vi "GDSAPI_CreateInterface.vi"(7 "KeepLvClassRefOpen(False)":bool, 8 "error in (no error)":errorcluster, 9 "ClassIcon(Random colors are used if not wired)":T1, 10 "CreateInterfaceType":T3, 11 "ProjectItemToCreateClassUnder":refnum<vi>) -> (0 "error out":errorcluster, 2 "LVClassLibraryRefnum":refnum<vi>, 3 "LvClassFileOut":path)   [LabVIEW 2020]
doc: "NOT Yet implemented"
uses:
  ClassProviders/Provider_LvNativeClass/ClassWriterNative_class/ClassWriterNative.lvclass
  ClassProviders/Common/LvIcon_class/GDSLvIcon_ClassColorTypes.ctl
  ClassProviders/Common/CommonVIs/CommonVIs_AttributeDataType.ctl
  ClassProviders/Common/String/GDSString_AccessScopeModifierType.ctl
  ClassProviders/Common/CommonVIs/CommonVIs_AttributeType.ctl
  ClassProviders/Provider_BaseClassInterface/ClassWriter_class/InterfaceMethodsToCreate.ctl
  ClassProviders/Provider_BaseClassInterface/ClassWriter_class/ClassWriter.lvclass
  ClassProviders/Provider_BaseClassInterface/CreateInterfaceData.ctl
  GDSAPI_SubVIs/GDSAPI_ClassIcon.ctl
  GDSAPI_SubVIs/GDSAPI_ClassIconType.ctl
  GDSAPI_CreateInterfaceType.ctl
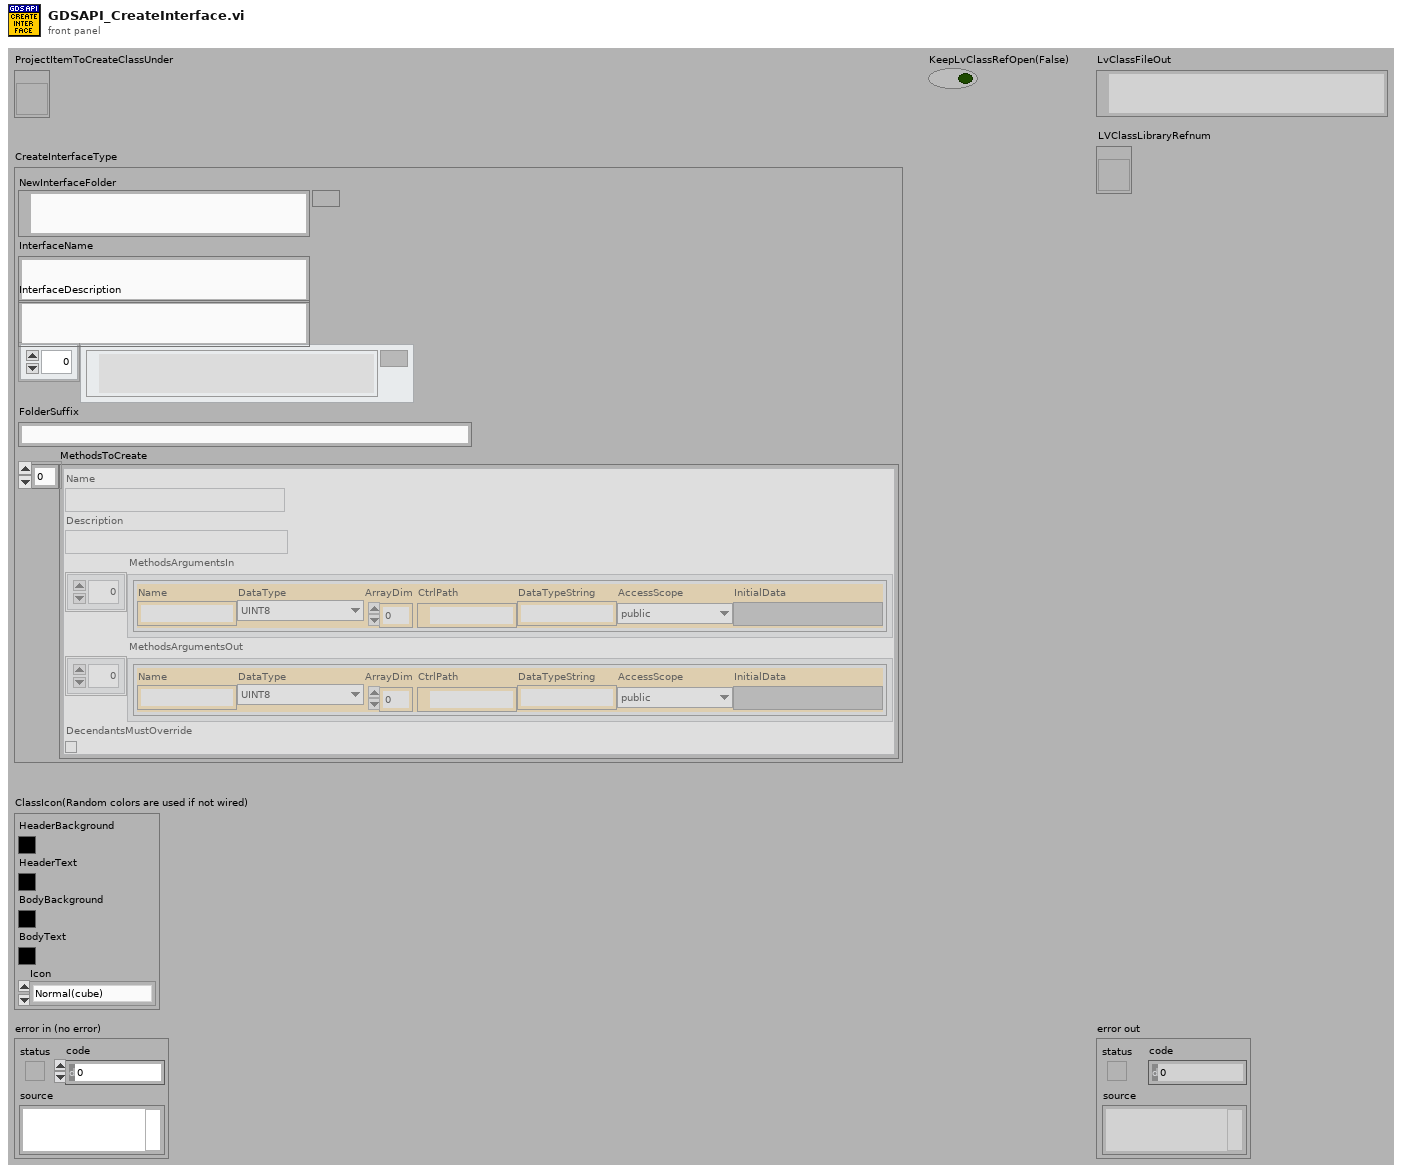
[diagram p1: front panel]
types:
  T1 = typedef "GDSAPI_ClassIcon.ctl" = cluster{"HeaderBackground":u32, "HeaderText":u32, "BodyBackground":u32, "BodyText":u32, "Icon":T2}
  T2 = typedef "GDSAPI_ClassIconType.ctl" = enum16{"Normal(cube)", "Actor", "Message", "Interface"}
  T3 = typedef "GDSAPI_CreateInterfaceType.ctl" = cluster{"NewInterfaceFolder":path, "InterfaceName":string, "InterfaceDescription":string, "ParentInterfacesFilePath":path[], "FolderSuffix":string, "MethodsToCreate":T4[]}
  T4 = typedef "ClassWriter.lvclass/InterfaceMethodsToCreate.ctl" = cluster{"Name":string, "Description":string, "MethodsArgumentsIn":T5[], "MethodsArgumentsOut":T5[], "DecendantsMustOverride":bool}
  T5 = typedef "CommonVIs_AttributeType.ctl" = cluster{"Name":string, "DataType":T6, "ArrayDim":i32, "CtrlPath":path, "DataTypeString":string, "AccessScope":T7, "InitialData":variant}
  T6 = typedef "CommonVIs_AttributeDataType.ctl" = enum16{"UINT8", "INT8", "UINT16", "INT16", "UINT32", "INT32", "UINT64", "INT64", "SGL", "DBL", "EXT", "CSG", "CDB", "CXT", "TimeStamp", "STRING", "PATH", "BOOL", "ENUM", "RefNum", "VIRefNum", "LabVIEW Class", "Cluster", "Variant", "TypeDef", "Waveform", "LabVIEW Object", "Other", "void", "Set", "Map"}
  T7 = typedef "GDSString_AccessScopeModifierType.ctl" = enum16{"public", "private", "protected", "internal"}
  T8 = typedef "ClassWriter.lvclass/CreateInterfaceData.ctl" = cluster{"InterfaceName":string, "InterfaceFolder":path, "InterfaceDescription":string, "FolderSuffix":string, "MethodsToCreate":T4[], "ParentInterfaces":path[]}
  T9 = typedef "GDSLvIcon_ClassColorTypes.ctl" = cluster{"Frame":u32, "Header Text Color":u32, "Header Background":u32, "BodyBackgroundPublic":u32, "BodyBackgroundProtected":u32, "BodyBackgroundPrivate":u32, "Body Text Color":u32, "Frame thickness":u8, "ProtectedPrivateSame":bool, "Icon Header Size":u8, "Font Compression":enum16{"Auto", "On", "Off"}, "CapitalOnly":bool}
  T10 = cluster{"Colors":T9, "LibraryIcon":cluster{"LibraryIcon":string, "HeaderRows(1)":u8}}
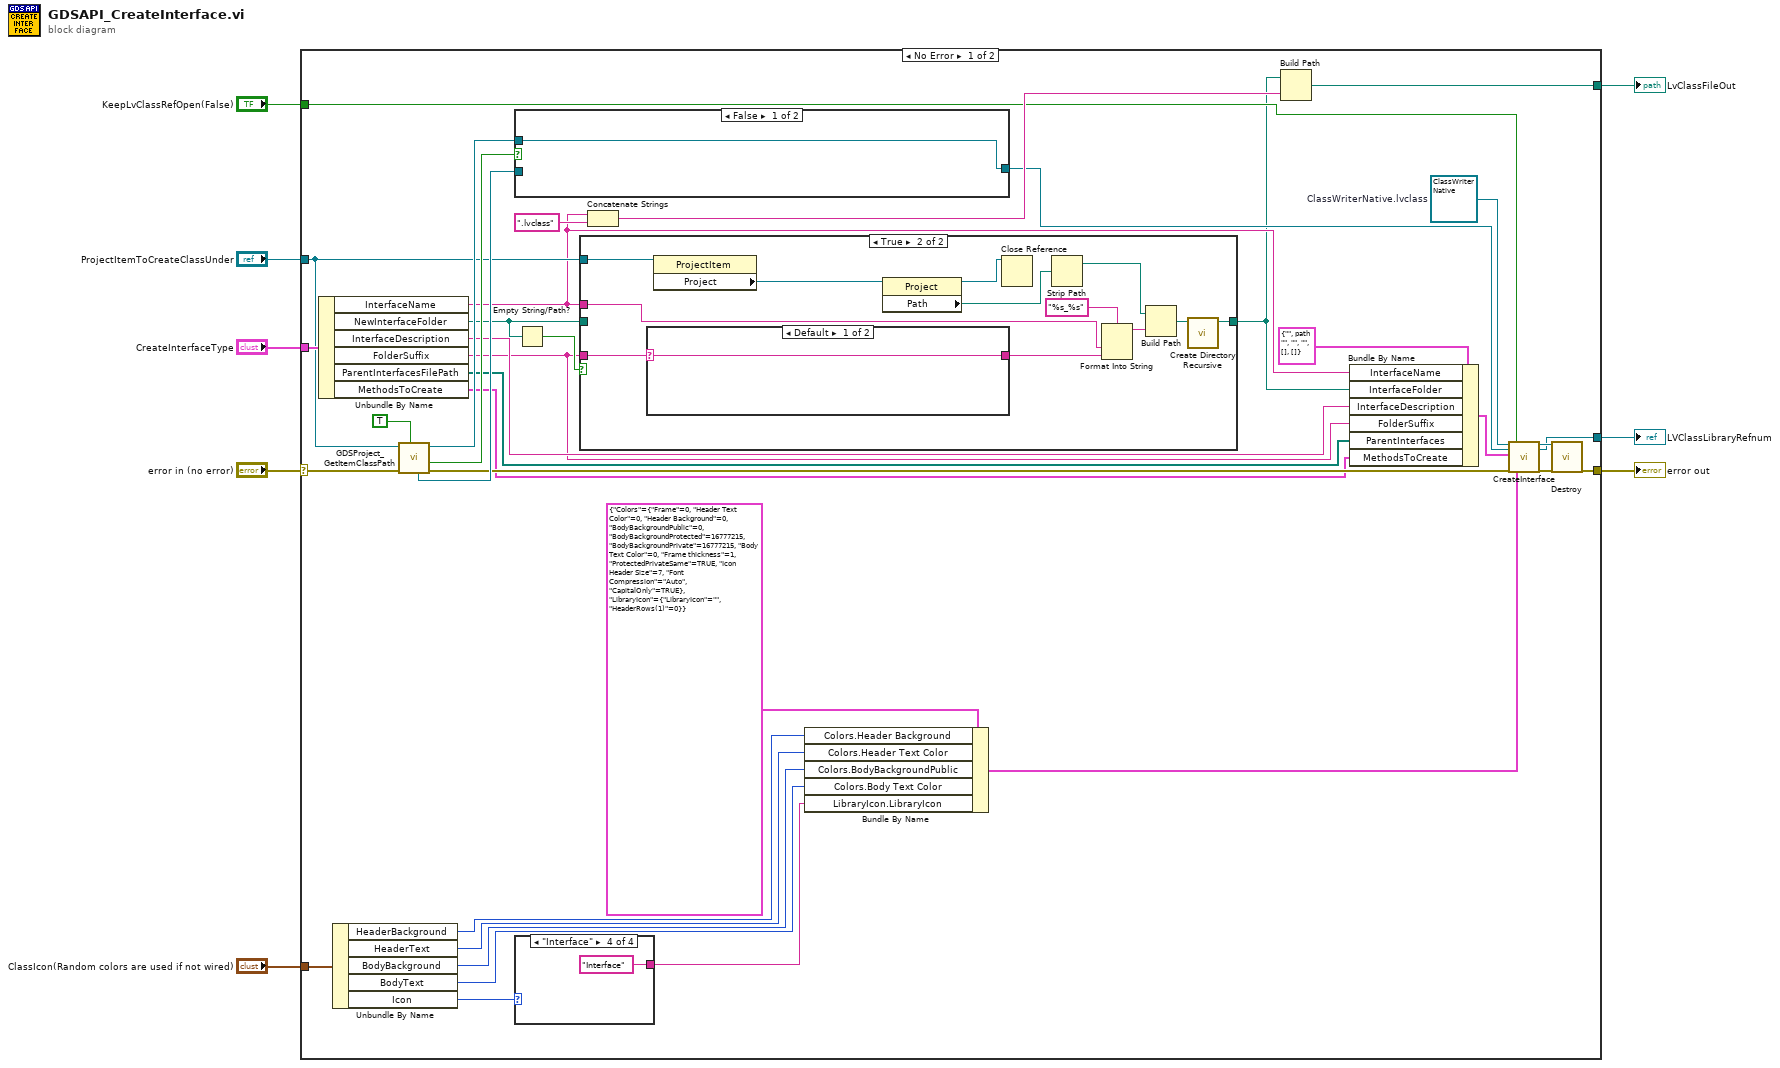
[diagram p0: block diagram]
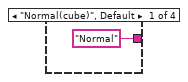
[diagram p2: hidden frame]
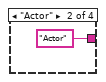
[diagram p3: hidden frame]
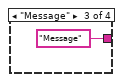
[diagram p4: hidden frame]
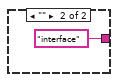
[diagram p6: hidden frame]
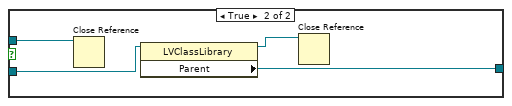
[diagram p7: hidden frame]
diagram:
  n1 = case shown="No Error" "error in (no error)" {
    selector: "error in (no error)" -> [w12 w70]
    tunnel: [w21 _] -> w8
    tunnel: [w41 w70] -> w7
    tunnel: "CreateInterfaceType" -> [w40 _]
    tunnel: "ProjectItemToCreateClassUnder" -> [w37 _]
    tunnel: "ClassIcon(Random colors are used if not wired)" -> [w35 _]
    tunnel: [w26 _] -> w3
    tunnel: "KeepLvClassRefOpen(False)" -> [w20 _]
    frame No Error {
      w25 = refnum<class "ClassWriterNative.lvclass"> refnum  # ClassWriterNative.lvclass
      n2 = Unbundle By Name(w40) -> ("InterfaceName"=w16:string, "NewInterfaceFolder"=w38:path, "InterfaceDescription"=w15:string, "FolderSuffix"=w10:string, "ParentInterfacesFilePath"=w11:path[], "MethodsToCreate"=w9:T4[])
      n3 = Unbundle By Name(w35) -> ("HeaderBackground"=w34:u32, "HeaderText"=w33:u32, "BodyBackground"=w32:u32, "BodyText"=w31:u32, "Icon"=w30:T2)
      n4 = call "GDSProject_GetItemClassPath.vi"("ReturnRefToClass(False)"=TRUE, "error in"=w12, "ProjectItemRefIn"=w37) -> ("error out"=w24:errorcluster, "LvCLassFound"=w44:bool, "ProjectItemRefOut"=w43:refnum<vi>, "LvClassRef"=w42:refnum<vi>)  [unwired: 3 in, 2 out]
      n5 = case shown="False" w44 {
        tunnel: w43 -> [w65 w69]
        tunnel: [w65 w67] -> w18
        tunnel: w42 -> [_ w68]
        frame False {
        }
        frame True {
          n6 = Close Reference(reference=w69) -> ()  [unwired: 1 in, 1 out]
          n7 = property class="LVClassLibrary"(reference=w68) -> (reference out=w66:refnum<vi>, "Parent"=w67:refnum<vi>)  [unwired: 1 in, 1 out]
          n8 = Close Reference(reference=w66) -> ()  [unwired: 1 in, 1 out]
        }
      }
      n9 = case shown="\"Interface\"" w30 {
        tunnel: ["Normal" ("LibraryIcon.LibraryIcon") "Actor" "Message" "Interface"] -> w29
        frame "Normal(cube)", Default {
        }
        frame "Actor" {
        }
        frame "Message" {
        }
        frame "Interface" {
        }
      }
      n10 = Empty String/Path?(string/path=w38) -> (empty?=w39:bool)
      n11 = case shown="True" w39 {
        tunnel: w38 -> [w50 _]
        tunnel: [w50 w54] -> w14
        tunnel: w37 -> [_ w62]
        tunnel: w16 -> [_ w52]
        tunnel: w10 -> [_ w51]
        frame False {
        }
        frame True {
          n12 = case shown="Default" w51 {
            selector: w51 -> [w63 _]
            tunnel: [w63 "interface" ("format string")] -> w53
            frame Default {
            }
            frame "" {
            }
          }
          n13 = property class="ProjectItem"(reference=w62) -> ("Project"=w61:refnum<vi>)  [unwired: 1 in, 2 out]
          n14 = property class="Project"(reference=w61) -> (reference out=w59:refnum<vi>, "Path"=w60:path)  [unwired: 1 in, 1 out]
          n15 = Close Reference(reference=w59) -> ()  [unwired: 1 in, 1 out]
          n16 = Strip Path(path=w60) -> (stripped path=w55:path)  [unwired: 1 out]
          n17 = Format Into String(format string="%s_%s", w52, w53) -> (resulting string=w57:string)  [unwired: 2 in, 1 out]
          n18 = Build Path(base path=w55, name or relative path=w57) -> (appended path=w56:path)
          n19 = call <vilib>:"Create Directory Recursive.vi"("directory"=w56) -> ("directory copy"=w54:path)  [unwired: 4 in, 2 out]
        }
      }
      n20 = Concatenate Strings(w16, ".lvclass" ("string")) -> (w27:string)
      n21 = Bundle By Name(cluster=T10 {"Colors"={"Frame"=0, "Header Text Color"=0, "Header Background"=0, "BodyBackgroundPublic"=0, "BodyBackgroundProtected"=16777215, "BodyBackgroundPrivate"=16777215, "Body Text Color"=0, "Frame thickness"=1, "ProtectedPrivateSame"=TRUE, "Icon Header Size"=7, "Font Compression"=enum."Auto", "CapitalOnly"=TRUE}, "LibraryIcon"={"LibraryIcon"="", "HeaderRows(1)"=0}} ("output cluster"), "Colors.Header Background"=w34, "Colors.Header Text Color"=w33, "Colors.BodyBackgroundPublic"=w32, "Colors.Body Text Color"=w31, "LibraryIcon.LibraryIcon"=w29) -> (w19:T10)
      n22 = Build Path(base path=w14, name or relative path=w27) -> (appended path=w26:path)
      n23 = Bundle By Name(cluster=T8 {"InterfaceName"="", "InterfaceFolder"=path "", "InterfaceDescription"="", "FolderSuffix"="", "MethodsToCreate"=[], "ParentInterfaces"=[]} ("CreateInterfaceData"), "InterfaceName"=w16, "InterfaceFolder"=w14, "InterfaceDescription"=w15, "FolderSuffix"=w10, "ParentInterfaces"=w11, "MethodsToCreate"=w9) -> (w13:T8)
      n24 = call-dynamic "CreateInterface.vi"("ClassWriterNative.lvclass"=w25, "ProjectTreePosition(String or Project Item Ref)"=w18, "CreateInterfaceData"=w13, "error in (no error)"=w24, "KeepLvClassRefOpen(False)"=w20, "HeaderToApply (take from VIRef or /use 2D-8bit header, Ignored if not wired)"=w19) -> ("ClassWriterNative.lvclass"=w23:refnum<class "ClassWriterNative.lvclass">, "LVClassLibraryRefnum"=w21:refnum<vi>, "error out"=w22:errorcluster)  [unwired: 11 in]
      n25 = call-dynamic "Destroy.vi"("ClassWriterNative"=w23, "error in (no error)"=w22) -> ("error out"=w41:errorcluster)  [unwired: 17 in]
    }
    frame Error {
    }
  }
  "error out" <- w7
  "LvClassFileOut" <- w3
  "LVClassLibraryRefnum" <- w8
